vi "to string.vi"(8 "error in":errorcluster, 11 "Thermo configuration":refnum<class "Thermo configuration.lvclass">) -> (0 "error out":errorcluster, 1 "data":string, 2 "version":string, 3 "Thermo configuration out":refnum<class "Thermo configuration.lvclass">)   [LabVIEW 2025, in "Thermo.lvlib" / "Thermo configuration.lvclass"]
doc: "Provides an interface for saving a module configuration to a file or other serialized data source. It is recommended that all children of this class store data in two sets--data required for its own initialization, and any data required for parent initialization--and that each implementation uses the <b>Call Parent Method</b> primitive to serialize parent information.Copyright 2017 National Instruments Corporation\n\nLicensed under the Apache License, Version 2.0 (the \"License\"); you may not use this file except in compliance with the License. You may obtain a copy of the License at http://www.apache.org/licenses/LICENSE-2.0\nUnless required by applicable law or agreed to in writing, software distributed under the License is distributed on an \"AS IS\" BASIS, WITHOUT WARRANTIES OR CONDITIONS OF ANY KIND, either express or implied. See the License for the specific language governing permissions and limitations under the License."
uses:
  Thermo configuration.lvclass
  C:/Users/Public/Documents/Sandia National Labs/TSS Plugin/Abstract Engine.lvlibp/Plugin/Abstract/Instrument configuration/Instrument configuration.lvclass
  Thermo configuration.lvclass/Thermo configuration.ctl
  Read Thermo Setting.vi
  Users/Public/Documents/Sandia National Labs/TSS Plugin/Abstract Engine.lvlibp/Plugin/Abstract/Instrument configuration/Read Instrument Setting.vi
  Users/Public/Documents/Sandia National Labs/TSS Plugin/Abstract Engine.lvlibp/Plugin/Abstract/Instrument configuration/Instrument configuration.lvclass
  Users/Public/Documents/Sandia National Labs/TSS Plugin/CEF.lvlibp/serializable configuration/CEF_serializable configuration.lvclass
  Users/Public/Documents/Sandia National Labs/TSS Plugin/CEF.lvlibp
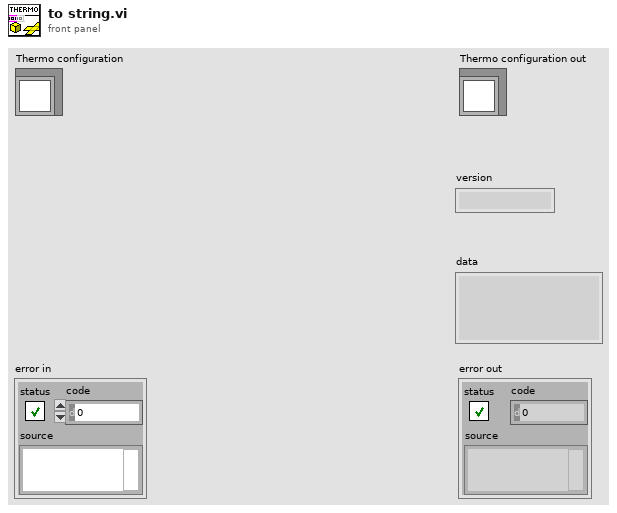
[diagram p1: front panel]
types:
  T1 = typedef "Thermo.lvlib/Thermo configuration.lvclass/Thermo Setting.ctl" = cluster{"Numeric":dbl, "Combo":string, "String":string, "Boolean":bool}
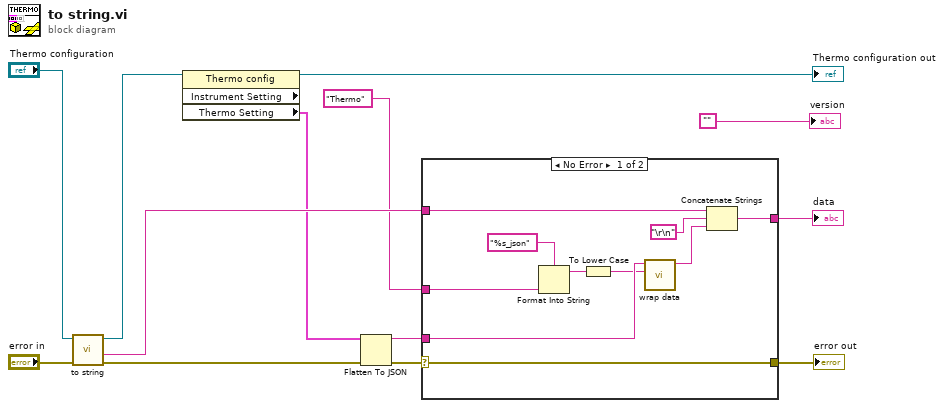
[diagram p0: block diagram]
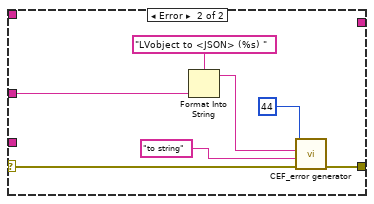
[diagram p2: hidden frame]
diagram:
  n1 = call-parent "to string.vi"("error in"="error in", "Instrument configuration"="Thermo configuration") -> ("error out"=w4:errorcluster, "data"=w8:string, "Instrument configuration out"=w11:refnum<class "Thermo configuration.lvclass">)  [unwired: 6 in, 1 out]
  n2 = property class="Thermo config" props=["Instrument Setting", "Thermo Setting"](reference=w11) -> (reference out=→"Thermo configuration out":refnum<class "Thermo configuration.lvclass">, "Thermo Setting"=w2:T1)  [unwired: 1 in, 2 out]
  n3 = Flatten To JSON(anything=w2, error in (no error)=w4) -> (JSON string=w9:string, 11:w10:errorcluster)  [unwired: 1 in]
  n4 = case shown="No Error" w10 {
    selector: w10 -> [w23 w28]
    tunnel: [w23 w27] -> w6
    tunnel: w9 -> [w21 _]
    tunnel: w8 -> [w20 _]
    tunnel: [w18 _] -> w7
    tunnel: "Thermo" ("additional identifier") -> [w14 w24]
    frame No Error {
      n5 = Format Into String(format string="%s_json" ("additional identifier"), w14) -> (resulting string=w16:string)  [unwired: 2 in, 1 out]
      n6 = To Lower Case(string=w16) -> (all lower case string=w15:string)
      n7 = call "wrap data.vi"("identifier"=w15, "data to wrap"=w21) -> ("wrapped data"=w22:string)  [unwired: 9 in]
      n8 = Concatenate Strings(w20, "\r\n", w22) -> (w18:string)
    }
    frame Error {
      n9 = Format Into String(format string="LVobject to <JSON> (%s) " ("message"), w24) -> (resulting string=w25:string)  [unwired: 2 in, 1 out]
      n10 = call "CEF_error generator.vi"("error in"=w28, "source"="to string" ("message"), "append error message"=w25, "error code (0)"=44) -> ("error out"=w27:errorcluster)  [unwired: 5 in]
    }
  }
  "error out" <- w6
  "data" <- w7
  "version" <- ""
